vi "Init.vi"(3 "Container State":T3, 4 "Previous State":variant, 5 "Previous Version":T2) -> (2 "Current State":T1)   [LabVIEW 2021, in "myRIO MSP.xctl"]
uses:
  <vilib>/myRIO/Common/Instrument Driver Framework/Utilities/xctls/myRIO MSP/myRIO MSP.xctl
  <vilib>/myRIO/Common/Instrument Driver Framework/Utilities/xctls/myRIO MSP/State.ctl
  <vilib>/_xctls/Container State.ctl
  <vilib>/_xctls/Version.ctl
  <vilib>/_xctls/XControlSupport.lvlib
panel:
  in  "Default Indicator State":T1
  in  "Default Control State":T1
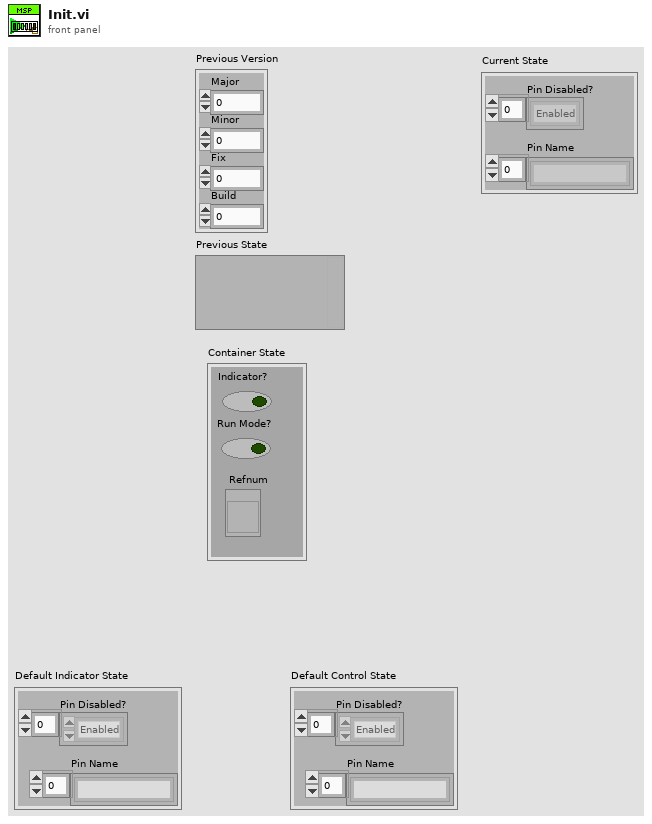
[diagram p1: front panel]
types:
  T1 = typedef "myRIO MSP.xctl/State.ctl" = cluster{"Pin Disabled?":enum8{"Enabled", "Disabled", "Disabled and Grayed Out"}[], "Pin Name":string[]}
  T2 = typedef "XControlSupport.lvlib/Version.ctl" = cluster{"Major":u16, "Minor":u16, "Fix":u16, "Build":u16}
  T3 = typedef "XControlSupport.lvlib/Container State.ctl" = cluster{"Indicator?":bool, "Run Mode?":bool, " Refnum":refnum<vi>}
  T4 = enum8{"Enabled", "Disabled", "Disabled and Grayed Out"}[]
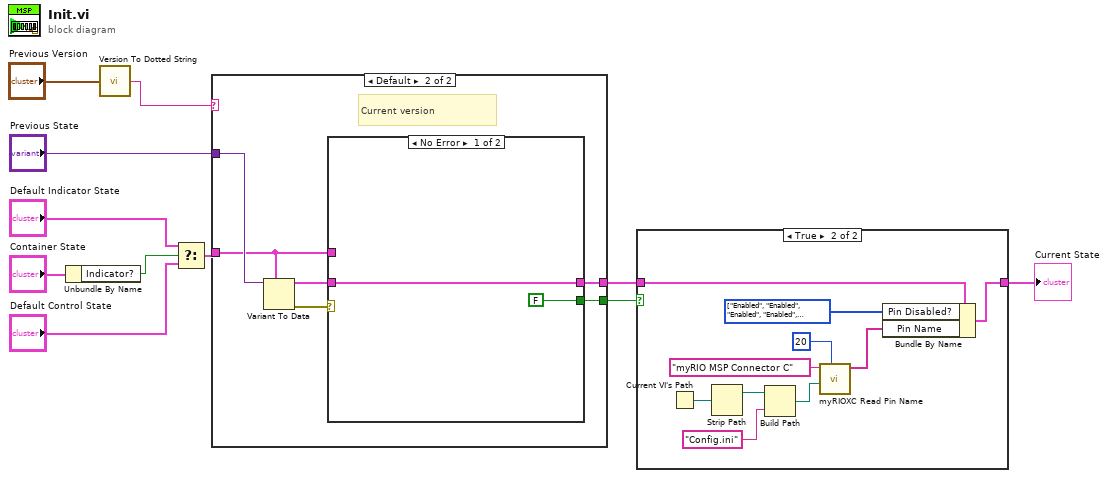
[diagram p0: block diagram]
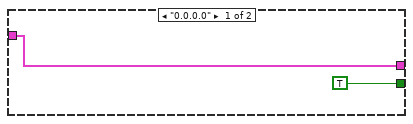
[diagram p3: hidden frame]
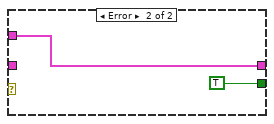
[diagram p4: hidden frame]
diagram:
  n1 = Unbundle By Name("Container State") -> ("Indicator?"=w7:bool)
  n2 = call <vilib>:"Version To Dotted String.vi"("Version"="Previous Version") -> ("String Version"=w4:string)
  n3 = Select(t="Default Indicator State", s=w7, f="Default Control State") -> (s? t:f=w6:T1)
  n4 = case shown="Default" w4 {
    tunnel: "Previous State" -> [_ w19]
    tunnel: [w13 w15] -> w3
    tunnel: w6 -> [w13 w16]
    tunnel: [TRUE w14] -> w1
    frame "0.0.0.0" {
    }
    frame Default {
      # "Current version"
      n5 = Variant To Data(type=w16, Variant=w19) -> (data=w17:T1, error out=w18:errorcluster)  [unwired: 1 in]
      n6 = case shown="No Error" w18 {
        tunnel: w17 -> [w21 _]
        tunnel: [w21 w23] -> w15
        tunnel: w16 -> [_ w23]
        tunnel: [FALSE TRUE] -> w14
        frame No Error {
        }
        frame Error {
        }
      }
    }
  }
  n7 = case shown="True" w1 {
    tunnel: w3 -> [w24 w34]
    tunnel: [w24 w33] -> w2
    frame False {
    }
    frame True {
      w32 = T4 [enum."Enabled", enum."Enabled", enum."Enabled", enum."Enabled", enum."Enabled", enum."Enabled", enum."Enabled", enum."Enabled", enum."Enabled", enum."Enabled", enum."Enabled", enum."Enabled", enum."Enabled", enum."Enabled", enum."Enabled", enum."Enabled", enum."Enabled", enum."Enabled", enum."Enabled", enum."Enabled", enum."Enabled", enum."Enabled", enum."Enabled", enum."Enabled", enum."Enabled", enum."Enabled", enum."Enabled", enum."Enabled", enum."Enabled", enum."Enabled", enum."Enabled", enum."Enabled", enum."Enabled", enum."Enabled"] items=["Enabled", "Disabled", "Disabled and Grayed Out"] ("Disabled?")
      n8 = Current VI's Path() -> (path=w25:path)
      n9 = Strip Path(path=w25) -> (stripped path=w27:path)  [unwired: 1 out]
      n10 = Build Path(base path=w27, name or relative path="Config.ini") -> (appended path=w26:path)
      n11 = call <vilib>:"myRIOXC Read Pin Name.vi"("Size"=20, "Path"=w26, "Connector"="myRIO MSP Connector C") -> ("Default Names"=w29:string[])  [unwired: 7 in, 1 out]
      n12 = Bundle By Name(cluster=w34, "Pin Disabled?"=w32, "Pin Name"=w29) -> (w33:T1)
    }
  }
  "Current State" <- w2
